vi "ODE Solver main_2.vi"(5 "data":variant, 7 "ODE F(X,t)":refnum<vi>, 8 "error in (no error)":errorcluster, 10 "simulation parameters":T1={"Initial Time"=0.0, "Final Time"=10.0, "Time Step"=0.1, "Absolute Tolerance"=0.001, "Relative Tolerance"=0.001, "Continuous Solver"=enum."Runge-Kutta 45 (variable)", "Discrete Time Step"=1.0, "Minimum Time Step"=1e-08, "Maximum Time Step"=1.0, "Initial Time Step"=0.01} {"Initial Time Step" min=0.0; "Maximum Time Step" min=0.0}, 11 "x0":dbl[](array[numeric])) -> (0 "error out":errorcluster, 2 "output":dbl[](array[numeric]), 3 "times":dbl[](array[numeric]))   [LabVIEW 2012]
doc: "Solves ordinary differential equations with initial conditions of the following form: X'=F(X,t). You must manually select the polymorphic instance to use."
uses:
  <vilib>/Simulation/Utility/Implementation/Shared/SIM Diagram Parameters.ctl
  <vilib>/Simulation/Implementation/Shared/SIM Continuous Solvers.ctl
  Synthetic_Jet_VIs/Lumped Element Model/SJ_ODE_Data.ctl
  Utilities/fluid_properties/fluid_types.ctl
  Synthetic_Jet_VIs/Lumped Element Model/LEM_Solution_Controls.ctl
  Synthetic_Jet_VIs/Lumped Element Model/Model.ctl
  Synthetic_Jet_VIs/Lumped Element Model/Fourier_Series.ctl
  Utilities/fluid_properties/fluid_properties.ctl
  <vilib>/Analysis/baseanly.llb/Scale 1D.vi
  <vilib>/Analysis/NI_AALPro.lvlib
  <vilib>/Analysis/NI_AALBase.lvlib
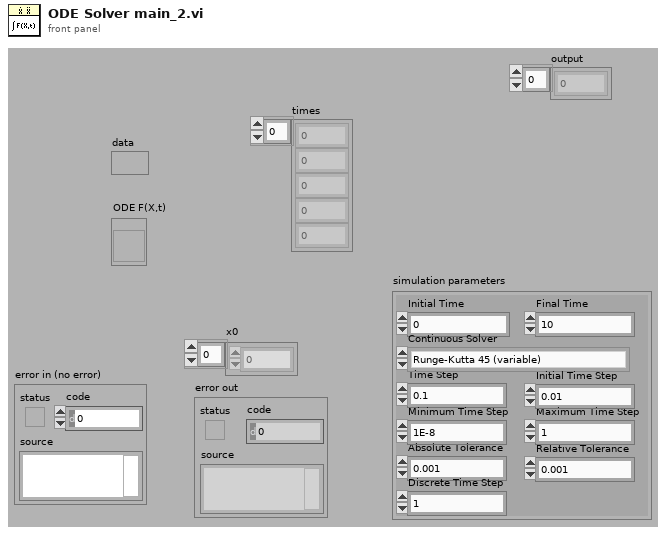
[diagram p1: front panel]
types:
  T1 = typedef "SIM Diagram Parameters.ctl" = cluster{"Initial Time":dbl, "Final Time":dbl, "Time Step":dbl, "Absolute Tolerance":dbl, "Relative Tolerance":dbl, "Continuous Solver":T2, "Discrete Time Step":dbl, "Minimum Time Step":dbl, "Maximum Time Step":dbl, "Initial Time Step":dbl}
  T2 = typedef "SIM Continuous Solvers.ctl" = enum16{"Runge-Kutta 1 (Euler)", "Runge-Kutta 2", "Runge-Kutta 3", "Runge-Kutta 4", "Runge-Kutta 23 (variable)", "Runge-Kutta 45 (variable)", "BDF (variable)", "Adams-Moulton (variable)", "Rosenbrock (variable)", "Discrete States Only"}
  T3 = typedef "SIM simulation data.ctl" = cluster{"continuous integrator":T4, "initial time":dbl, "final time":dbl, "step size":dbl, "proposed step size":dbl, "max step size":dbl, "min step size":dbl, "discrete time step":dbl, "max step ratio":dbl, "Diag Eval Stage":T5, "Substep Index":i32, "Timestep Index":dbl, "simulation time":dbl, "current timestep base":dbl, "proposed step time":dbl, "absolute tolerance":dbl, "relative tolerance":dbl, "step accepted?":bool, "step complete?":bool, "Halt?":bool, "reset integrator?":bool, "machine epsilon":dbl, "min float":dbl, "error":errorcluster, "Method Order":u32, "Finished Late [i-1]":bool, "Discrete step?":bool, "NaN and Inf check?":bool, "Final Timestep Index":dbl, "(maj+disc)or(init)?":bool, "Full Solver Reset":bool, "Execution Mode":T6, "check vector sizes?":bool, "solver handles zc?":bool, "Simulation Registry":T7, "variable step solver?":bool, "First Substep?":bool, "Continuous States?":bool}
  T4 = typedef "SIM integration method.ctl" = enum16{"RK 1 (Euler)", "Linearizer", "State Query", "Trim Eval", "Adams", "RK 3", "RK 4", "RK 45", "BDF", "RK 2", "RK 23", "Rosenbrock", "Discrete States Only"}
  T5 = typedef "SIM diagram eval stage.ctl" = enum16{"Init", "Minor Substep", "Major Substep", "Final"}
  T6 = typedef "SIMSCR Execution Mode.ctl" = enum16{"Simulate to Completion", "Single Time-Step Simulation (Fixed Step Only)"}
  T7 = typedef "SIM Simulation Registry.ctl" = cluster{"Current Idx":i32, "Node Tags":string[], "Node Headers":T8[], "Node Data":T9[], "Cont State data":T11, "DiscreteInfo":T13, "Disc State data":T14, "Registry Error":T15, "ZC Indices":i32[]}
  T8 = typedef "SIM Registry Node Header.ctl" = cluster{"Input Width":i32, "Disc ID":i32, "Num Cont St":i32, "Cont St Idx":i32, "Num Disc St":i32, "Disc St Idx":i32, "Output Width":i32}
  T9 = typedef "SIM Registry Node Record.ctl" = cluster{"Node Data":dbl[], "Node Outputs":dbl[], "Z.C. Signals":dbl[], "Z.C. Trigger Types":T10[]}
  T10 = typedef "SIM trigger type.ctl" = enum16{"rising", "falling", "either", "none"}
  T11 = typedef "SIM solver state data.ctl" = cluster{"inputs":dbl[], "outputs":dbl[], "reset":dbl[], "lower limits":dbl[], "upper limits":dbl[], "limit types":T12[], "reset types":T10[], "initial conditions":dbl[], "reset I.C.":dbl[], "limited?":bool[], "State Names":string[]}
  T12 = typedef "SIM limit type.ctl" = enum16{"upper", "lower", "both", "none"}
  T13 = typedef "SIM discrete data.ctl" = cluster{"tick period (sec)":dbl, "time (ticks)":i32, "fire?":bool[], "registry":cluster{"period (sec)":dbl[], "skew (sec)":dbl[], "period (tick)":i32[], "skew (tick)":i32[]}, "discrete \nblocks?":bool, "steps per tick":dbl, "steps to tick":dbl, "discrete \ntick?":bool}
  T14 = typedef "SIM Discrete state data.ctl" = cluster{"Disc States":dbl[], "State Names":string[]}
  T15 = typedef "SIM Simulation Registry Error.ctl" = cluster{"Error Block ID":i32, "code":i32}
  T16 = typedef "SJ_ODE_Data.ctl" = cluster{"Fluid Properties":cluster{"Fluid":T17, "Temperature (K)":dbl, "Pressure (Pa)":dbl}, "SJ Geometry":cluster{"Do (mm)":dbl, "Ho (mm)":dbl, "Dc (mm)":dbl, "Hc (mm)":dbl}, "Solution Controls":T18, "Misc Data":cluster{"Freq jet":dbl, "Coefficients":dbl[], "Nat Frequ":dbl, "Ku":dbl, "Scale":dbl, "Fourier Series":T20, "Km":dbl, "Kr":dbl}, "Thermo and Transport Properties":T21, "LEM Output Data":cluster{"X":dbl[][], "times":dbl[], "|X|":dbl, "PA X":dbl}}
  T17 = typedef "fluid_types.ctl" = enum16{"Air", "Water"}
  T18 = typedef "LEM_Solution_Controls.ctl" = cluster{"Simulation":enum16{"Sinusoidal", "Fourier Series"}, "Fixed Parameter":enum16{"Pressure", "Displacement"}, "Model":T19, "# time steps":i32, "# periods":i32, "Tolerance":dbl, "STFT periods":i32}
  T19 = typedef "Model.ctl" = enum16{"Martin", "Tang", "Gallas", "Persoon"}
  T20 = typedef "Fourier_Series.ctl" = cluster{"Amp":dbl, "Phase":dbl}[]
  T21 = typedef "fluid_properties.ctl" = cluster{"nu":dbl, "c":dbl, "Pr":dbl, "Cp":dbl, "Cv":dbl, "gamma":dbl, "mu":dbl, "rho":dbl}
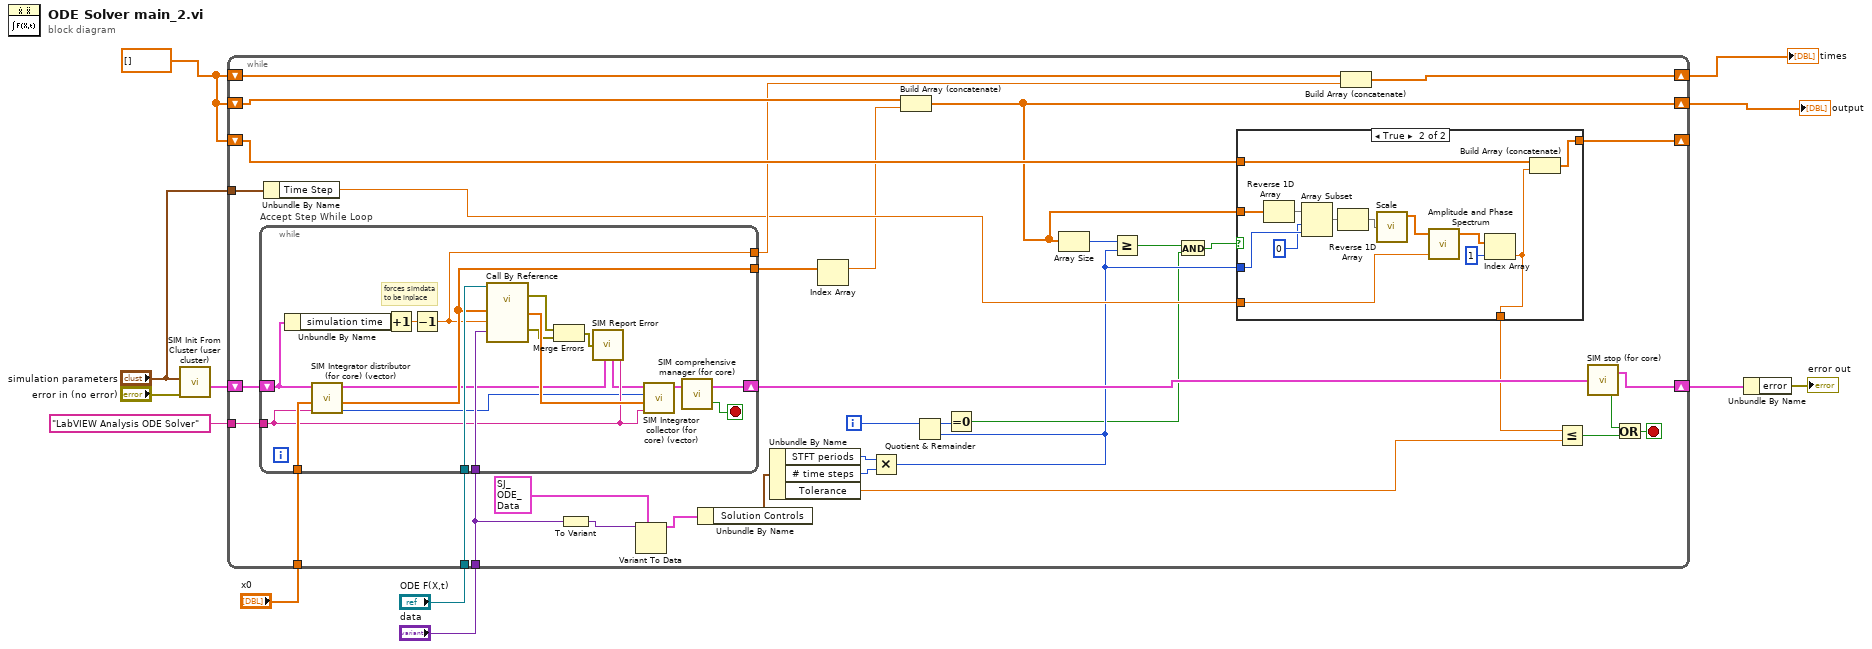
[diagram p0: block diagram]
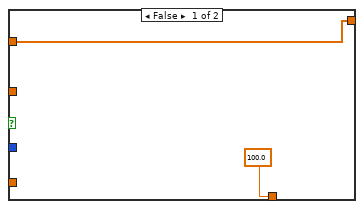
[diagram p2: hidden frame]
diagram:
  w3 = dbl[] []
  n1 = call <vilib>:"SIM Init From Cluster (user cluster).vi"("errorin"="error in (no error)", "Sim Params"="simulation parameters") -> ("Simulation data out"=w6:T3)  [unwired: 5 in]
  n2 = while "Simulation While Loop" {
    shift-right: [w47] -> w12
    shift-left: w6 -> [w32]
    tunnel: "ODE F(X,t)" -> [w46]
    tunnel: "data" -> [w40]
    tunnel: "x0" -> [w45]
    tunnel: "LabVIEW Analysis ODE Solver" -> [w44]
    shift-right: [w43] -> w2
    shift-left: w3 -> [w42]
    shift-right: [w13] -> w1
    shift-left: w3 -> [w35]
    shift-right: [w24] -> _
    shift-left: w3 -> [w27]
    tunnel: "simulation parameters" -> [w23]
    i -> [w20]
    stop <- w29 stop-if-true
    n3 = while "Accept Step While Loop" {
      shift-right: [w71] -> w48
      shift-left: w32 -> [w70]
      tunnel: w46 -> [w81]
      tunnel: w40 -> [w76]
      tunnel: w45 -> [w74]
      tunnel: [w75] -> w41
      tunnel: [w67] -> w22
      tunnel: w44 -> [w73]
      stop <- w82 stop-if-true
      # "forces simdata\nto be inplace"
      n4 = Unbundle By Name(w70) -> ("simulation time"=w69:dbl)
      n5 = call <vilib>:"SIM Integrator distributor (for core) (vector).vi"("DNL_Simulation CallChain"=w73, "initial condition"=w74, "Simulation data"=w70) -> ("width"=w72:i32, "output"=w75:dbl[], "Simulation data out"=w64:T3)  [unwired: 6 in]
      n6 = Increment(x=w69) -> (x+1=w68:dbl)
      n7 = Decrement(x=w68) -> (x-1=w67:dbl)
      n8 = call-by-ref "?"(reference=w81, "data"=w76, "t"=w67, "x"=w75) -> (error out=w80:errorcluster, 0:"error out"=w77:errorcluster, "f'(x)"=w78:dbl[])  [unwired: 1 in, 1 out]
      n9 = Merge Errors(w80, w77) -> (w79:errorcluster)
      n10 = call <vilib>:"SIM Report Error.vi"("error in (no error)"=w79, "Simulation data"=w64, "DNL_Simulation CallChain"=w73) -> ("Simulation data out"=w65:T3)  [unwired: 6 in]
      n11 = call <vilib>:"SIM Integrator collector (for core) (vector).vi"("DNL_Simulation CallChain"=w73, "input"=w78, "width"=w72, "Simulation data"=w65) -> ("Simulation data out"=w66:T3)  [unwired: 7 in]
      n12 = call <vilib>:"SIM comprehensive manager (for core).vi"("Simulation data"=w66) -> ("step complete?"=w82:bool, "Simulation data out"=w71:T3)  [unwired: 1 in]
    }
    n13 = Unbundle By Name(w23) -> ("Time Step"=w21:dbl)
    n14 = To Variant(anything=w40) -> (Variant=w39:variant)
    n15 = Variant To Data(type=T16 {"Fluid Properties"={"Fluid"=enum."Air", "Temperature (K)"=300.0, "Pressure (Pa)"=100000.0}, "SJ Geometry"={"Do (mm)"=5.0, "Ho (mm)"=8.0, "Dc (mm)"=40.0, "Hc (mm)"=6.5}, "Solution Controls"={"Simulation"=enum."Sinusoidal", "Fixed Parameter"=enum."Pressure", "Model"=enum."Tang", "# time steps"=1, "# periods"=340, "Tolerance"=0.0, "STFT periods"=0}, "Misc Data"={"Freq jet"=0.0, "Coefficients"=[], "Nat Frequ"=0.0, "Ku"=0.0, "Scale"=0.0, "Fourier Series"=[], "Km"=0.0, "Kr"=0.0}, "Thermo and Transport Properties"={"nu"=0.0, "c"=0.0, "Pr"=0.0, "Cp"=0.0, "Cv"=0.0, "gamma"=0.0, "mu"=0.0, "rho"=0.0}, "LEM Output Data"={"X"=[], "times"=[], "|X|"=0.0, "PA X"=0.0}} ("ODE Data"), Variant=w39) -> (data=w37:T16)  [unwired: 1 in, 1 out]
    n16 = Unbundle By Name(w37) -> ("Solution Controls"=w36:T18)
    n17 = Unbundle By Name(w36) -> ("STFT periods"=w34:i32, "# time steps"=w33:i32, "Tolerance"=w31:dbl)
    n18 = Index Array(array=w41) -> (element=w14:dbl)  [unwired: 1 in]
    n19 = Multiply(x=w34, y=w33) -> (x*y=w19:i32)
    n20 = Build Array (concatenate)(w35, w14) -> (w13:dbl[])
    n21 = Quotient & Remainder(x=w20, y=w19) -> (x-y*floor(x/y)=w18:i32)  [unwired: 1 out]
    n22 = Equal To 0?(x=w18) -> (x = 0?=w16:bool)
    n23 = Array Size(array=w13) -> (size(s)=w28:i32)
    n24 = Greater Or Equal?(x=w28, y=w19) -> (x >= y?=w17:bool)
    n25 = And(x=w17, y=w16) -> (x .and. y?=w15:bool)
    n26 = case shown="True" w15 {
      tunnel: w13 -> [_ w63]
      tunnel: w19 -> [_ w61]
      tunnel: w21 -> [_ w59]
      tunnel: [w50 w57] -> w24
      tunnel: w27 -> [w50 w56]
      tunnel: [100.0 w55] -> w25
      frame False {
      }
      frame True {
        n27 = Reverse 1D Array(array=w63) -> (reversed array=w62:dbl[])
        n28 = Array Subset(array=w62, index=0, length=w61) -> (w53:dbl[])
        n29 = Reverse 1D Array(array=w53) -> (reversed array=w52:dbl[])
        n30 = call-poly <vilib>:"Scale.vi"("X"=w52) -> ("Y=(X-offset)/scale"=w51:dbl[])  [unwired: 3 out]
        n31 = call <vilib>:"Amplitude and Phase Spectrum.vi"("dt"=w59, "Signal (V)"=w51) -> ("Amp Spectrum Mag (Vrms)"=w54:dbl[])  [unwired: 1 in, 2 out]
        n32 = Index Array(array=w54, index=1) -> (element=w55:dbl)
        n33 = Build Array (concatenate)(w56, w55) -> (w57:dbl[])
      }
    }
    n34 = Build Array (concatenate)(w42, w22) -> (w43:dbl[])
    n35 = Less Or Equal?(x=w25, y=w31) -> (x <= y?=w26:bool)
    n36 = call <vilib>:"SIM stop (for core).vi"("Simulation data"=w48) -> ("Simulation data out"=w47:T3, "stop simulation?"=w30:bool)
    n37 = Or(x=w30, y=w26) -> (x .or. y?=w29:bool)
  }
  "times" <- w2
  "output" <- w1
  n38 = Unbundle By Name(w12) -> ("error"=→"error out":errorcluster)
